vi "Reset Theme.vi"(8 "error in":errorcluster) -> (0 "error out":errorcluster)   [LabVIEW 2021, in "Theme.lvclass"]
doc: "Reset the global theme for the application - this unloads the global theme that will be used and uses the default theme or input from a VI\n\n<b>Code Developed By:</b> +\nDaniel Coons +\nhttps://github.com/danielcoons/tsc-pop-up"
uses:
  Theme.lvclass
  Popup/PopUp Theme Global.vi
  Theme.lvclass/Theme.ctl
  Popup/Popup.lvclass
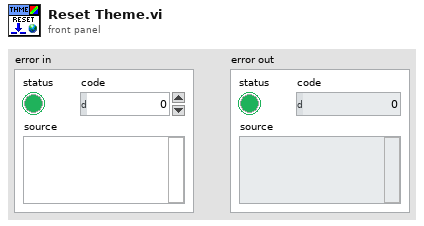
[diagram p1: front panel]
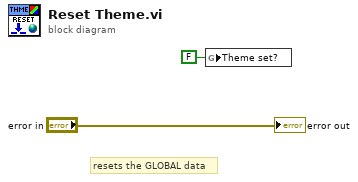
[diagram p0: block diagram]
diagram:
  # "resets the GLOBAL data"
  n1 = global write "PopUp Theme Global.vi" "Theme set?"(FALSE ("Theme set?")) -> ()
  "error out" <- "error in"
